vi "Init Drive Motors.vi"() -> ()   [LabVIEW 2017]
uses:
  <vilib>/Rock Robotics/WPI/RobotDrive/WPI_RobotDriveOpen4MotorWithExistingMotors.vi
panel:
  out "error out":errorcluster
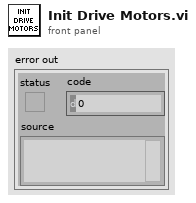
[diagram p1: front panel]
types:
  T1 = typedef "WPI_MotorControlDeviceRef.ctl" = cluster{"DeviceStatus":errorcluster, "Type":T2, "PWM":cluster{"PWM Channel":T3, "DeadBand":T4}, "CAN":cluster{"Device Number":u8, "SetOutput VI Ref":variant, "GetOutput VI Ref":variant, "Enable VI Ref":variant, "Disable VI Ref":variant, "Data":variant}, "Invert":bool, "DIO PWM":cluster{"PWM \"Enable\" Channel":T3, "DIOChannel":T5, "PWM Rate":dbl}}
  T2 = typedef "WPI_MotorControlType.ctl" = enum16{"PWM", "CAN", "DIO PWM"}
  T3 = typedef "FPGA_DIOPWMChannel.ctl" = enum8{"PWM 0", "PWM 1", "PWM 2", "PWM 3", "PWM 4", "PWM 5", "PWM 6", "PWM 7", "PWM 8", "PWM 9", "PWM MXP 0", "PWM MXP 1", "PWM MXP 2", "PWM MXP 3", "PWM MXP 4", "PWM MXP 5", "PWM MXP 6", "PWM MXP 7", "PWM MXP 8", "PWM MXP 9", "Invalid"}
  T4 = typedef "WPI_PWMDeadband.ctl" = cluster{"Name":string, "maxPositivePwm":i32, "minPositivePwm":i32, "centerPwm":i32, "maxNegativePwm":i32, "minNegativePwm":i32, "angularRange":u16}
  T5 = typedef "FPGA_DIOChannel.ctl" = enum8{"DIO 0", "DIO 1", "DIO 2", "DIO 3", "DIO 4", "DIO 5", "DIO 6", "DIO 7", "DIO 8", "DIO 9", "DIO MXP 0", "DIO MXP 1", "DIO MXP 2", "DIO MXP 3", "DIO MXP 4", "DIO MXP 5", "DIO MXP 6", "DIO MXP 7", "DIO MXP 8", "DIO MXP 9", "DIO MXP 10", "DIO MXP 11", "DIO MXP 12", "DIO MXP 13", "DIO MXP 14", "DIO MXP 15", "SPI Port CS1", "SPI Port CS2", "SPI Port CS3", "SPI Port MISO", "SPI Port MOSI", "Invalid"}
  T6 = typedef "WPI_RobotDriveDevRef.ctl" = cluster{"DevStatus":errorcluster, "Motors[]":T1[], "Square Inputs":bool, "Max Output":dbl}
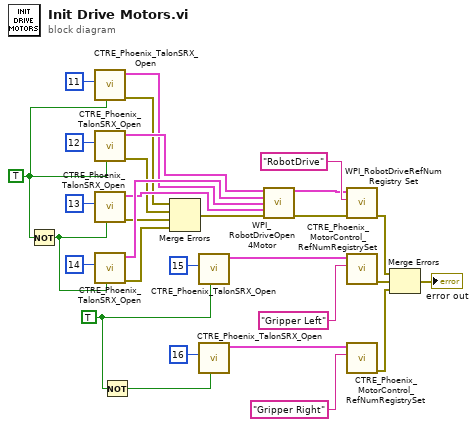
[diagram p0: block diagram]
diagram:
  w6 = TRUE ("Invert")
  w20 = TRUE ("Invert")
  n1 = Not(x=w20) -> (.not. x?=w19:bool)
  n2 = call "CTRE_Phoenix_TalonSRX_Open.vi"("Invert"=w20, "Device Number"=u8 11) -> ("error out"=w18:errorcluster, "CAN Talon SRX Ref"=w22:T1)  [unwired: 8 in]
  n3 = call "CTRE_Phoenix_TalonSRX_Open.vi"("Invert"=w20, "Device Number"=u8 12) -> ("error out"=w17:errorcluster, "CAN Talon SRX Ref"=w24:T1)  [unwired: 8 in]
  n4 = call "CTRE_Phoenix_TalonSRX_Open.vi"("Invert"=w19, "Device Number"=u8 13) -> ("error out"=w16:errorcluster, "CAN Talon SRX Ref"=w21:T1)  [unwired: 8 in]
  n5 = call "CTRE_Phoenix_TalonSRX_Open.vi"("Invert"=w19, "Device Number"=u8 14) -> ("error out"=w15:errorcluster, "CAN Talon SRX Ref"=w23:T1)  [unwired: 8 in]
  n6 = Not(x=w6) -> (.not. x?=w5:bool)
  n7 = Merge Errors(w18, w17, w16, w15) -> (w14:errorcluster)
  n8 = call "CTRE_Phoenix_TalonSRX_Open.vi"("Invert"=w6, "Device Number"=u8 15) -> ("CAN Talon SRX Ref"=w10:T1)  [unwired: 8 in, 1 out]
  n9 = call "CTRE_Phoenix_TalonSRX_Open.vi"("Invert"=w5, "Device Number"=u8 16) -> ("CAN Talon SRX Ref"=w8:T1)  [unwired: 8 in, 1 out]
  n10 = call-poly <vilib>:"WPI_RobotDriveOpen4Motor.vi"("Rear Left Motor Dev Ref"=w24, "Rear Right Motor Dev Ref"=w23, "Front Left Motor Dev Ref"=w22, "Front Right Motor Dev Ref"=w21, "error in (no error)"=w14) -> ("RobotDriveDevRef"=w26:T6, "error out"=w13:errorcluster)  [unwired: 9 in]
  n11 = call <vilib>:"WPI_RobotDriveRefNum Registry Set.vi"("error in (no error)"=w13, "refnum name"="RobotDrive", "RobotDriveDevRef"=w26) -> ("error out"=w4:errorcluster)  [unwired: 7 in, 1 out]
  n12 = call <vilib>:"CTRE_Phoenix_MotorControl_RefNumRegistrySet.vi"("refnum name"="Gripper Left", "PhoenixMotorControlDevRef"=w10) -> ("error out"=w3:errorcluster)  [unwired: 8 in, 1 out]
  n13 = call <vilib>:"CTRE_Phoenix_MotorControl_RefNumRegistrySet.vi"("refnum name"="Gripper Right", "PhoenixMotorControlDevRef"=w8) -> ("error out"=w2:errorcluster)  [unwired: 8 in, 1 out]
  n14 = Merge Errors(w4, w3, w2) -> (→"error out":errorcluster)
